vi "Attentionlayer_backpropagation.vi"(6 "Array":fxp<+/-,32,16>[](array[numeric])=[0.0, 0.0, 0.0, 0.0, 0.0, 0.0, 0.0, 0.0, 0.0, 0.0, 0.0, 0.0, 0.0, 0.0, 0.0, 0.0, 0.0, 0.0, 0.0, 0.0, 0.0, 0.0, 0.0, 0.0, 0.0, 0.0, 0.0, 0.0, 0.0, 0.0, 0.0, 0.0, 0.0, 0.0, 0.0, 0.0, 0.0, 0.0, 0.0, 0.0, 0.0, 0.0, 0.0, 0.0, 0.0, 0.0, 0.0, 0.0, 0.0, 0.0], 7 "Array 2":fxp<+/-,32,16>[](array[numeric])=[0.0, 0.0, 0.0, 0.0, 0.0, 0.0, 0.0, 0.0, 0.0, 0.0, 0.0, 0.0, 0.0, 0.0, 0.0, 0.0, 0.0, 0.0, 0.0, 0.0, 0.0, 0.0, 0.0, 0.0, 0.0], 9 "Numeric":fxp<+/-,32,16>, 10 "Numeric 2":fxp<+/-,32,16>, 11 "Numeric 3":fxp<+/-,32,16>) -> ()   [LabVIEW 2020]
uses:
  <vilib>/rvi/interface/RandomDataEmulation/niFpgaRandomDataHandleErrors.vi
  <vilib>/rvi/DataTransferAndStorage/Container/XNode/niFpgaContainer.xnode
  <vilib>/rvi/interface/RandomDataEmulation/nirviRandomDataFpgaReadWriteTemplate.vi
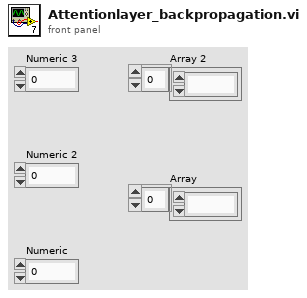
[diagram p1: front panel]
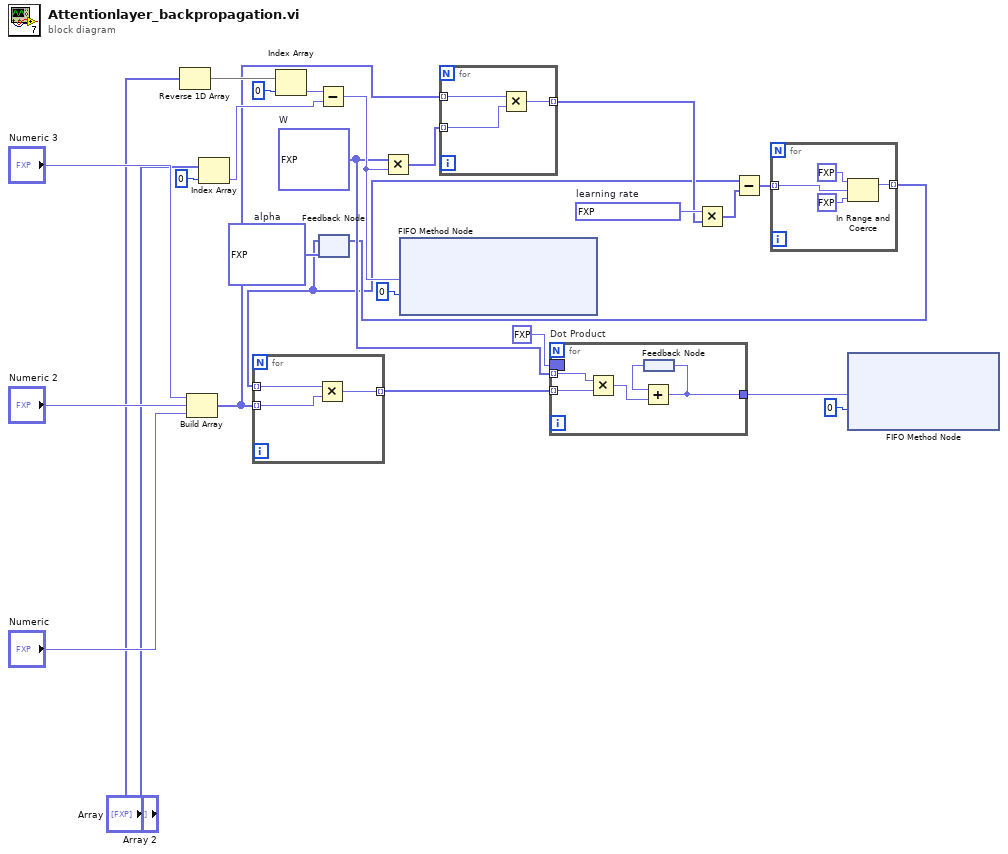
[diagram p0: block diagram]
diagram:
  w25 = fxp<+/-,32,16>[] [0.3330078125, 0.3330078125, 0.3330078125]  # W
  w19 = fxp<+/-,32,16> 0.899993896484375  # learning rate
  w20 = fxp<+/-,32,16>[] [0.3330078125, 0.3330078125, 0.3330078125]  # alpha
  n1 = Reverse 1D Array(array="Array") -> (reversed array=w7:fxp<+/-,32,16>[])
  n2 = Build Array("Numeric 3", "Numeric 2", "Numeric") -> (w1:fxp<+/-,32,16>[])
  n3 = Index Array(array="Array 2", index=0) -> (element=w5:fxp<+/-,32,16>)
  n4 = Index Array(array=w7, index=0) -> (element=w6:fxp<+/-,32,16>)
  n5 = Subtract(x=w6, y=w5) -> (x-y=w26:fxp<+/-,32,16>)
  n6 = feedback #1(w20) -> (w2:fxp<+/-,32,16>[])
  n7 = for {
    tunnel: [w29] -> w3 mode=indexing
    tunnel: w2 -> [w28] mode=indexing
    tunnel: w1 -> [w27] mode=indexing
    n8 = Multiply(x=w28, y=w27) -> (x*y=w29:fxp<+/-,32,16>)
  }
  n9 = Multiply(x=w25, y=w26) -> (x*y=w9:fxp<+/-,32,16>[])
  n10 = xnode ("FIFO Method Node")("Element"=w26, "Timeout"=0) -> ()  [unwired: 1 in, 2 out]
  n11 = for {
    tunnel: [w32] -> w10 mode=indexing
    tunnel: w1 -> [w31] mode=indexing
    tunnel: w9 -> [w30] mode=indexing
    n12 = Multiply(x=w31, y=w30) -> (x*y=w32:fxp<+/-,64,32>)
  }
  n13 = for "Dot Product" {
    tunnel: [w36] -> w4
    tunnel: w3 -> [w35] mode=indexing
    tunnel: w25 -> [w34] mode=indexing
    border: fxp<+/-,32,16> 0.0 -> [_]
    n14 = Multiply(x=w34, y=w35) -> (x*y=w33:fxp<+/-,32,16>)
    n15 = feedback #2() -> (w37:fxp<+/-,32,16>)
    n16 = Add(x=w37, y=w33) -> (x+y=w36:fxp<+/-,32,16>)
    n17 = feedback-in #2(w36) -> ()
  }
  n18 = Multiply(x=w19, y=w10) -> (x*y=w11:fxp<+/-,32,16>[])
  n19 = Subtract(x=w2, y=w11) -> (x-y=w8:fxp<+/-,32,16>[])
  n20 = for {
    tunnel: w8 -> [w41] mode=indexing
    tunnel: [w38] -> w24 mode=indexing
    n21 = In Range and Coerce(upper limit=fxp<+/-,32,16> 1.0, x=w41, lower limit=fxp<+/-,32,16> 0.0) -> (coerced(x)=w38:fxp<+/-,32,16>)  [unwired: 1 out]
  }
  n22 = feedback-in #1(w24) -> ()
  n23 = xnode ("FIFO Method Node")("Element"=w4, "Timeout"=0) -> ()  [unwired: 1 in, 2 out]
